vi "UUT_CheckRule.vi"(8 "error in (no error)":errorcluster caption="错误输入（无错误）", 11 "UUT输入":T1) -> (0 "error out":errorcluster caption="错误输入（无错误）", 2 "CheckString":string, 3 "DataRuleOK？":bool)   [LabVIEW 2013, in "Settings-Style.lvlib"]
uses:
  Settings-Style.lvlib
  1_Ctl/DB_UUT.ctl
  1_ctl/Ctl-Color.ctl
panel:
  # "Style Settings"
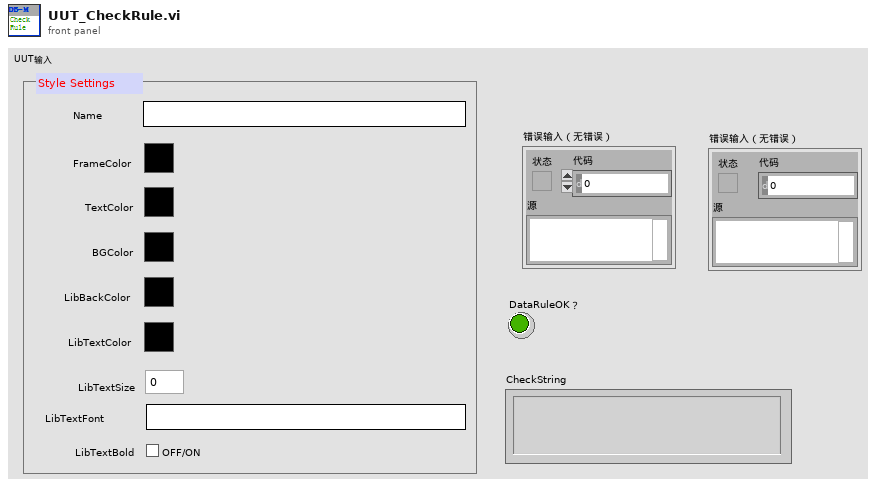
[diagram p1: front panel]
types:
  T1 = typedef "Settings-Style.lvlib/DB_UUT.ctl" = cluster{"Name":string, "FrameColor":T2, "TextColor":T2, "BGColor":T2, "LibBackColor":T2, "LibTextColor":T2, "LibTextSize":dbl, "LibTextFont":string, "LibTextBold":bool}
  T2 = typedef "Ctl-Color.ctl" = u32
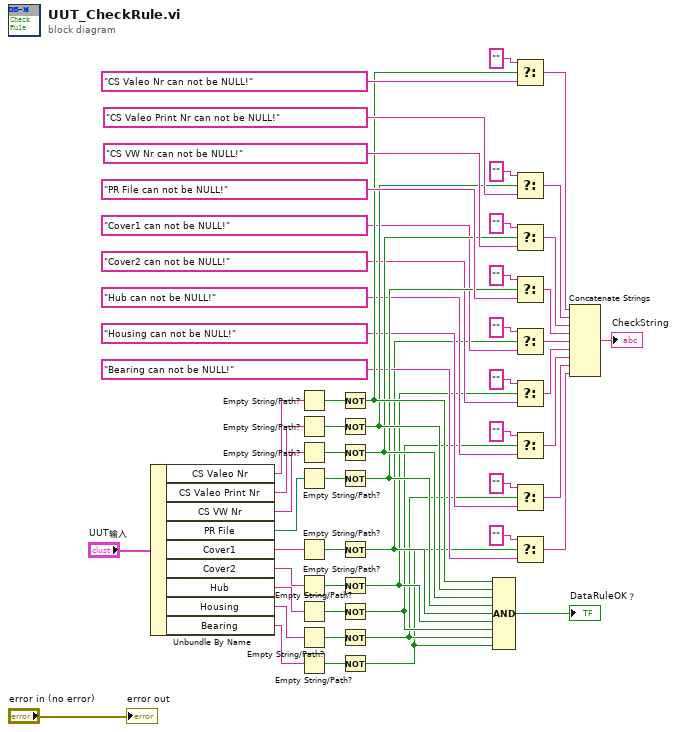
[diagram p0: block diagram]
diagram:
  n1 = Unbundle By Name("UUT输入") -> ("CS Valeo Nr"=w56:string, "CS Valeo Print Nr"=w41:string, "CS VW Nr"=w40:string, "PR File"=w39:path, "Cover1"=w25:string, "Cover2"=w24:string, "Hub"=w23:string, "Housing"=w22:string, "Bearing"=w21:string)
  n2 = Empty String/Path?(string/path=w56) -> (empty?=w55:bool)
  n3 = Empty String/Path?(string/path=w41) -> (empty?=w48:bool)
  n4 = Empty String/Path?(string/path=w40) -> (empty?=w47:bool)
  n5 = Empty String/Path?(string/path=w39) -> (empty?=w42:bool)
  n6 = Empty String/Path?(string/path=w25) -> (empty?=w30:bool)
  n7 = Empty String/Path?(string/path=w24) -> (empty?=w29:bool)
  n8 = Empty String/Path?(string/path=w23) -> (empty?=w28:bool)
  n9 = Empty String/Path?(string/path=w22) -> (empty?=w27:bool)
  n10 = Empty String/Path?(string/path=w21) -> (empty?=w26:bool)
  n11 = Not(x=w55) -> (.not. x?=w38:bool)
  n12 = Not(x=w48) -> (.not. x?=w36:bool)
  n13 = Not(x=w47) -> (.not. x?=w35:bool)
  n14 = Not(x=w42) -> (.not. x?=w34:bool)
  n15 = Not(x=w30) -> (.not. x?=w10:bool)
  n16 = Not(x=w29) -> (.not. x?=w9:bool)
  n17 = Not(x=w28) -> (.not. x?=w8:bool)
  n18 = Not(x=w27) -> (.not. x?=w7:bool)
  n19 = Not(x=w26) -> (.not. x?=w6:bool)
  n20 = Compound Arithmetic op=AND(w38, w36, w35, w34, w10, w9, w8, w7, w6) -> (→"DataRuleOK？":bool)
  n21 = Select(t="", s=w38, f="CS Valeo Nr can not be NULL!") -> (s? t:f=w54:string)
  n22 = Select(t="", s=w36, f="CS Valeo Print Nr can not be NULL!") -> (s? t:f=w33:string)
  n23 = Select(t="", s=w35, f="CS VW Nr can not be NULL!") -> (s? t:f=w32:string)
  n24 = Select(t="", s=w34, f="PR File can not be NULL!") -> (s? t:f=w31:string)
  n25 = Select(t="", s=w10, f="Cover1 can not be NULL!") -> (s? t:f=w5:string)
  n26 = Select(t="", s=w9, f="Cover2 can not be NULL!") -> (s? t:f=w4:string)
  n27 = Select(t="", s=w8, f="Hub can not be NULL!") -> (s? t:f=w3:string)
  n28 = Select(t="", s=w7, f="Housing can not be NULL!") -> (s? t:f=w2:string)
  n29 = Select(t="", s=w6, f="Bearing can not be NULL!") -> (s? t:f=w1:string)
  n30 = Concatenate Strings(w54, w33, w32, w31, w5, w4, w3, w2, w1) -> (→"CheckString":string)
  "error out" <- "error in (no error)"
